vi "CSM - Mark As Worker Module.vi"(9 "CSM Name":string) -> (2 "CSM Name(marked as worker)":string)   [LabVIEW 2020, in "Communicable State Machine.lvlib"]
doc: "Append '#' to CSM Name, to mark this module is a worker, who shares the same message queue with workers with the same name. A real name with uuid generated will be assigned to this CSM module.\n\n<b>Inputs:</b>\n - <b>CSM Name</b>: CSM module name.\n\n<b>Outputs:</b>\n - <b>CSM Name(marked as worker)</b>: CSM module name with '#' appended."
uses:
  Communicable State Machine.lvlib
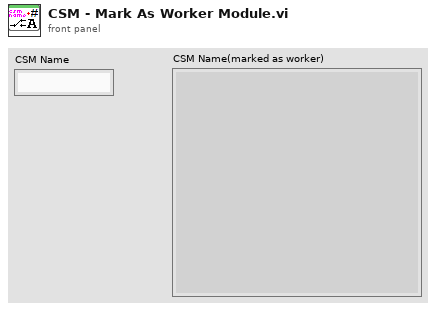
[diagram p1: front panel]
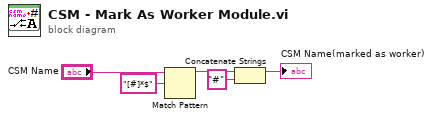
[diagram p0: block diagram]
diagram:
  n1 = Match Pattern(string="CSM Name", regular expression="[#]*$") -> (before substring=w3:string)  [unwired: 1 in, 3 out]
  n2 = Concatenate Strings(w3, "#" ("string")) -> (→"CSM Name(marked as worker)":string)
